vi "bmp_to_png_RECURSIVE.vi"() -> ()   [LabVIEW 2017]
panel:
  out "in":path
  in  "Compression (-1...9)":i32=-1 min=-1 max=9 step=1
  out "Current Index":i32
  out "out":path
  in  "Folder Path":path
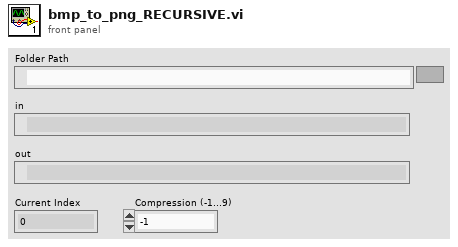
[diagram p1: front panel]
types:
  T1 = enum16{"open", "replace", "create", "open or create", "replace or create", "replace or create with confirmation"}
  T2 = typedef "imagedata.ctl" = cluster{"image type":i32, "image depth":i32, "image":u8[], "mask":u8[], "colors":u32[], "Rectangle":cluster{"left":i16, "top":i16, "right":i16, "bottom":i16}}
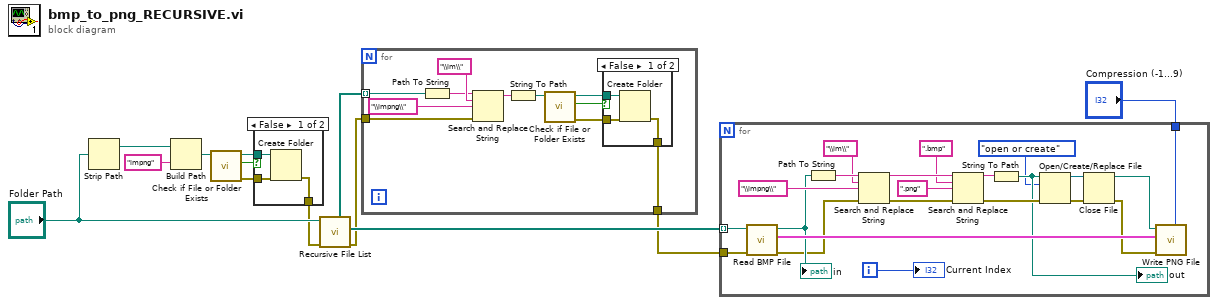
[diagram p0: block diagram]
diagram:
  n1 = Strip Path(path="Folder Path") -> (stripped path=w10:path)  [unwired: 1 out]
  n2 = Build Path(base path=w10, name or relative path="impng") -> (appended path=w8:path)
  n3 = call <vilib>:"Check if File or Folder Exists.vi"("path"=w8) -> ("error out"=w5:errorcluster, "file or folder exists?"=w7:bool, "dup path"=w6:path)  [unwired: 8 in]
  n4 = case shown="False" w7 {
    tunnel: w6 -> [w16 _]
    tunnel: w5 -> [w15 w17]
    tunnel: [w14 w17] -> w4
    frame False {
      n5 = Create Folder(path (use dialog)=w16, error in=w15) -> (error out=w14:errorcluster)  [unwired: 1 in, 2 out]
    }
    frame True {
    }
  }
  n6 = call <vilib>:"Recursive File List.vi"("error in (no error)"=w4, "Folder Path"="Folder Path") -> ("error out"=w2:errorcluster, "All Files in Dir"=w13:path[], "All Folders"=w3:path[])  [unwired: 5 in, 2 out]
  n7 = for {
    tunnel: w3 -> [w25] mode=indexing
    tunnel: w2 -> [w24]
    tunnel: [w18] -> w1
    n8 = Path To String(path=w25) -> (string=w26:string)
    n9 = Search and Replace String(input string=w26, search string="\\im\\", replace string="\\impng\\" ("replace string (\"\")"), error in=w24) -> (result string=w23:string)  [unwired: 4 in, 3 out]
    n10 = String To Path(string=w23) -> (path=w22:path)
    n11 = call <vilib>:"Check if File or Folder Exists.vi"("path"=w22) -> ("error out"=w19:errorcluster, "file or folder exists?"=w20:bool, "dup path"=w21:path)  [unwired: 8 in]
    n12 = case shown="False" w20 {
      tunnel: w21 -> [w31 _]
      tunnel: w19 -> [w30 w32]
      tunnel: [w29 w32] -> w18
      frame False {
        n13 = Create Folder(path (use dialog)=w31, error in=w30) -> (error out=w29:errorcluster)  [unwired: 1 in, 2 out]
      }
      frame True {
      }
    }
  }
  n14 = for {
    tunnel: w13 -> [w53] mode=indexing
    tunnel: "Compression (-1...9)" -> [w48]
    tunnel: w1 -> [w33]
    i -> [w49]
    n15 = call <vilib>:"Read BMP File.vi"("error in (no error)"=w33, "path to BMP file"=w53) -> ("error out"=w41:errorcluster, "image data"=w54:T2, "path"=w47:path)  [unwired: 7 in]
    "in" <- w47
    n16 = Path To String(path=w47) -> (string=w52:string)
    n17 = Search and Replace String(input string=w52, search string="\\im\\", replace string="\\impng\\" ("replace string (\"\")"), error in=w41) -> (result string=w46:string, error out=w43:errorcluster)  [unwired: 4 in, 2 out]
    n18 = Search and Replace String(input string=w46, search string=".bmp", replace string=".png" ("replace string (\"\")"), error in=w43) -> (result string=w42:string, error out=w40:errorcluster)  [unwired: 4 in, 2 out]
    n19 = String To Path(string=w42) -> (path=w38:path)
    "out" <- w38
    n20 = Open/Create/Replace File(file path (use dialog)=w38, error in=w40, operation (0:open)=T1."open or create") -> (refnum out=w39:refnum<file>, error out=w37:errorcluster)  [unwired: 3 in, 1 out]
    n21 = Close File(refnum=w39, error in=w37) -> (path=w35:path, error out=w36:errorcluster)
    n22 = call <vilib>:"Write PNG File.vi"("compression (default)"=w48, "error in (no error)"=w36, "image data"=w54, "path to PNG file"=w35) -> ()  [unwired: 6 in, 2 out]
    "Current Index" <- w49
  }
